vi "NewChoosePass.vi"(1 "IA State Input":T1={"our_robots"=[], "enemy_robots"=[], "balls"=[], "geometry"={"line_width"=0, "field_length"=0, "field_width"=0, "boundary_width"=0, "referee_width"=0, "goal_width"=0, "goal_depth"=0, "goal_wall_width"=0, "center_circle_radius"=0, "defense_radius"=0, "defense_stretch"=0, "free_kick_from_defense_dist"=0, "penalty_spot_from_field_line_dist"=0, "penalty_line_from_spot_dist"=0}, "IA Judge"={"stage"="", "command"="", "our_goalie_id"=0.0, "enemy_goalie_id"=0.0, "command enum"=enum."Halt", "Time"=enum."Azul"}, "Received Timestamp"=timestamp(0 s since 1904-01-01), "Events"={"Touch"=FALSE, "Ball out"=FALSE, "id touch"=0.0, "Ball out of \nVision"=FALSE, "Ball inside \nGoalie area"=FALSE, "Robot not responding"=FALSE, "Robots responding status"=[1.0, 1.0, 1.0, 1.0, 1.0, 1.0], "Enemy Ball \nPossession"=FALSE, "Pass State"=FALSE, "id end of pass"=0.0, "Kick"=FALSE, "Id ini Possession"=0.0, "Ball Possesion"=FALSE, "Id Possesion"=0.0, "Direct Kick"=FALSE, "2nd Strk Ativo"=FALSE}}) -> (0 "Receptor passe":enum16{"Auto", "2nd Striker", "Striker"}(ring))   [LabVIEW 2018]
uses:
  newpass/SSLView/Core/AI Input.ctl
  newpass/SSLView/Core/AI Robot.ctl
  newpass/SSLView/Intel/Functions Enum.ctl
  newpass/SSLView/Intel/AttackerStates.ctl
  newpass/SSLView/Path Planning/RRT/PathDests.ctl
  newpass/SSLView/Path Planning/RRT/PathDest.ctl
  newpass/SSLView/Core/AI Ball.ctl
  newpass/SSLView/Core/Field Size.ctl
  newpass/SSLView/Core/AI Judge.ctl
  newpass/SSLView/Intel/Command Enum.ctl
  newpass/SSLView/Util/Events/Events.ctl
panel:
  in  "x":dbl format="%#_13g"
  in  "y 3":dbl=0.4 format="%#_13g"
  in  "y 2":dbl=0.3 format="%#_13g"
  in  "y":dbl=0.3 format="%#_13g"
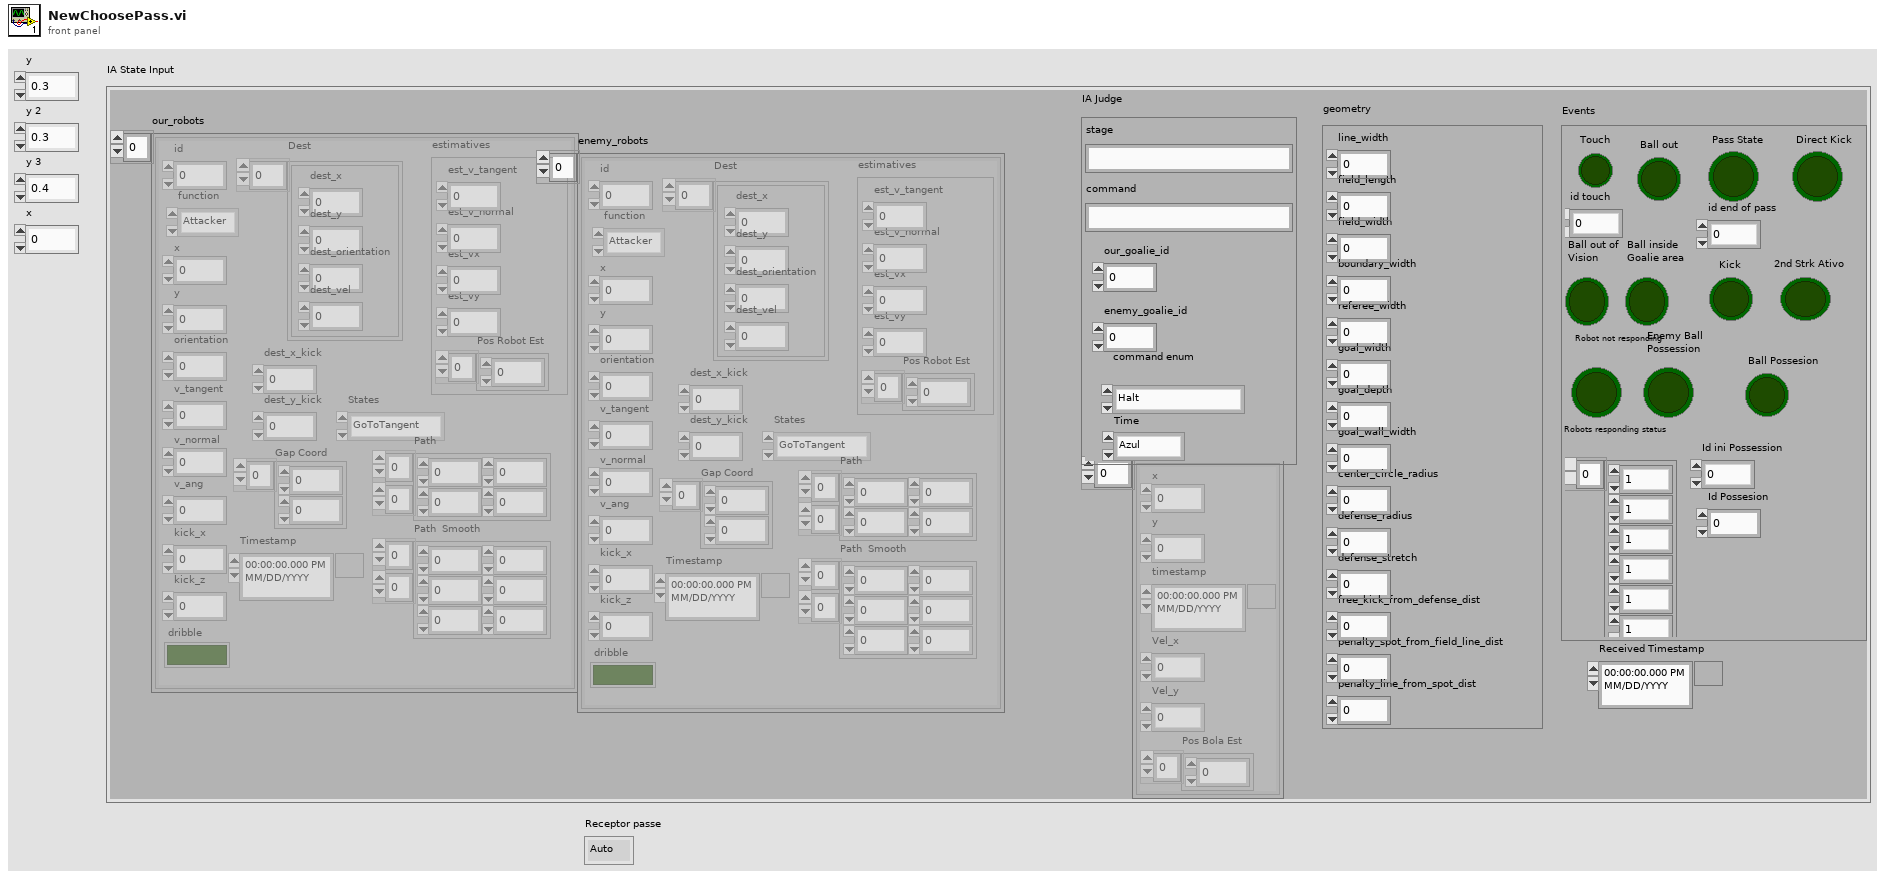
[diagram p1: front panel]
types:
  T1 = typedef "AI Input.ctl" = cluster{"our_robots":T2[], "enemy_robots":T2[], "balls":T7[], "geometry":T8, "IA Judge":T9, "Received Timestamp":timestamp, "Events":T11}
  T2 = typedef "AI Robot.ctl" = cluster{"id":u32, "function":T3, "x":dbl, "y":dbl, "orientation":dbl, "v_tangent":dbl, "v_normal":dbl, "v_ang":dbl, "kick_x":dbl, "kick_z":dbl, "dribble":bool, "Timestamp":timestamp, "estimatives":cluster{"est_v_tangent":dbl, "est_v_normal":dbl, "est_vx":dbl, "est_vy":dbl, "Pos Robot Est":dbl[]}, "dest_x_kick":dbl, "dest_y_kick":dbl, "Gap Coord":dbl[], "States":T4, "Path ":dbl[][], "Path  Smooth":dbl[][], "Dest":T5}
  T3 = typedef "Functions Enum.ctl" = enum16{"2nd Striker", "Attacker", "Goalie", "Defender", "Striker", "Goto 0", "Dummy", "Kicker", "ZigZag 0", "ZigZag 1", "ZigZag 2", "ZigZag 3", "ZigZag 4", "ZigZag 5", "ZigZag 6", "ZigZag 7", "ZigZag 8", ""}
  T4 = typedef "AttackerStates.ctl" = enum16{"Pass", "GoToTangent", "BallGetting", "GoToKick", ""}
  T5 = typedef "PathDests.ctl" = T6[]
  T6 = typedef "PathDest.ctl" = cluster{"dest_x":dbl, "dest_y":dbl, "dest_orientation":dbl, "dest_vel":dbl}
  T7 = typedef "AI Ball.ctl" = cluster{"x":dbl, "y":dbl, "timestamp":timestamp, "Vel_x":dbl, "Vel_y":dbl, "Pos Bola Est":dbl[]}
  T8 = typedef "Field Size.ctl" = cluster{"line_width":u32, "field_length":u32, "field_width":u32, "boundary_width":u32, "referee_width":u32, "goal_width":u32, "goal_depth":u32, "goal_wall_width":u32, "center_circle_radius":u32, "defense_radius":u32, "defense_stretch":u32, "free_kick_from_defense_dist":u32, "penalty_spot_from_field_line_dist":u32, "penalty_line_from_spot_dist":u32}
  T9 = typedef "AI Judge.ctl" = cluster{"stage":string, "command":string, "our_goalie_id":dbl, "enemy_goalie_id":dbl, "command enum":T10, "Time":enum16{"Azul", "Amarelo"}}
  T10 = typedef "Command Enum.ctl" = enum16{"Halt", "Stop", "Force Start", "PKA Normal Start", "Prepare Kickoff Ally", "PKE Normal Start", "Prepare Kickoff Enemy", "Prepare Penalty Ally", "PPA Normal Start", "Prepare Penalty Enemy", "PPE Normal Start", "Direct Free Enemy", "Direct Free Ally", "Indirect Free Enemy", "Indirect Free Ally", "Timeout Enemy", "Timeout Ally", "Goal Enemy", "Goal Ally", "Ball Placement Enemy", "Ball Placement Ally", "Normal Half Time", "Extra Time Break", "Extra Half Time", "None", "Post Game"}
  T11 = typedef "Events.ctl" = cluster{"Touch":bool, "Ball out":bool, "id touch":dbl, "Ball out of \nVision":bool, "Ball inside \nGoalie area":bool, "Robot not responding":bool, "Robots responding status":dbl[], "Enemy Ball \nPossession":bool, "Pass State":bool, "id end of pass":dbl, "Kick":bool, "Id ini Possession":dbl, "Ball Possesion":bool, "Id Possesion":dbl, "Direct Kick":bool, "2nd Strk Ativo":bool}
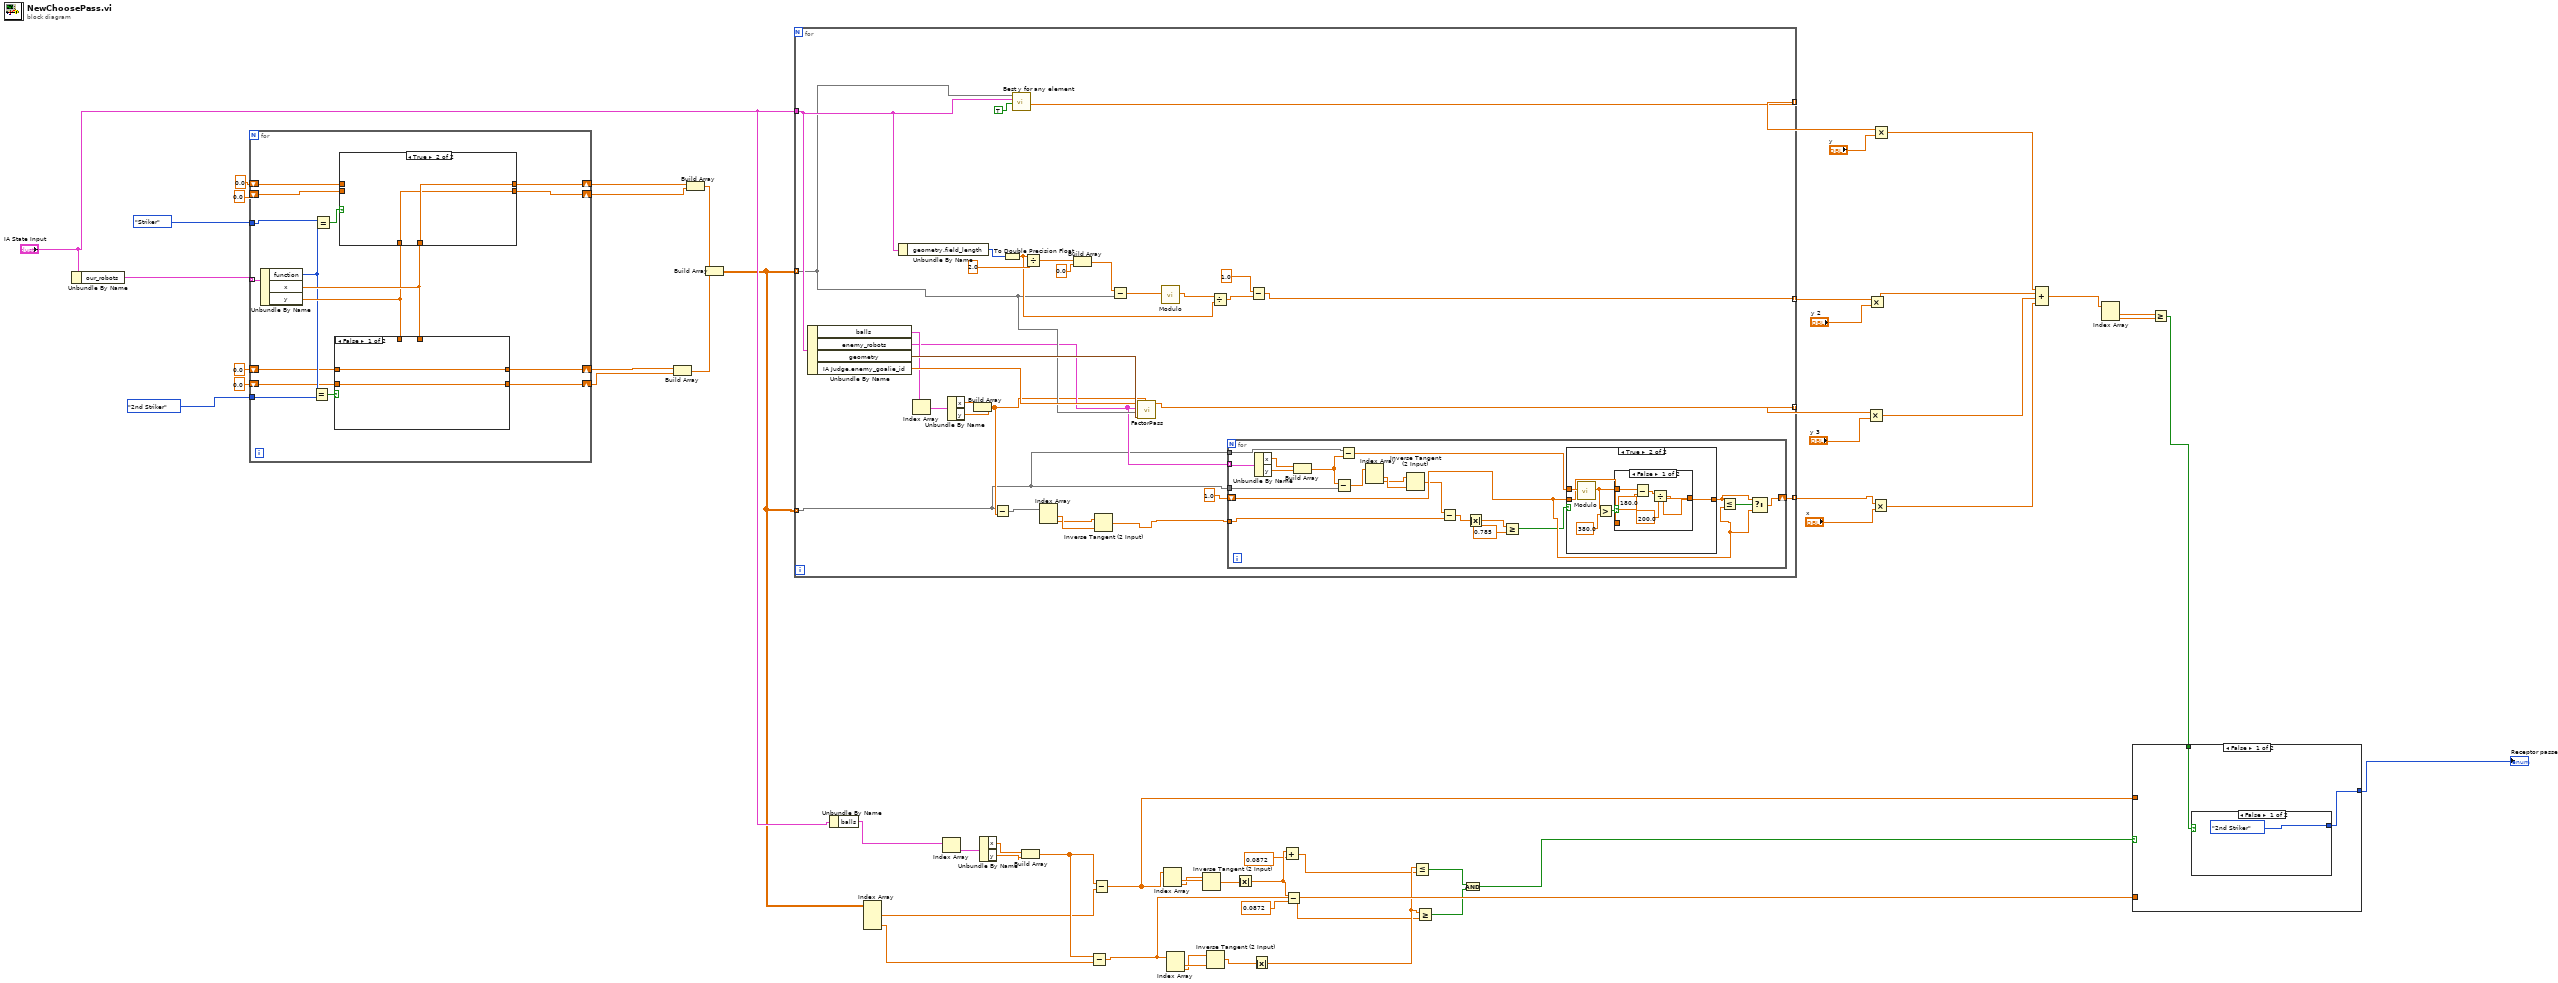
[diagram p0: block diagram]
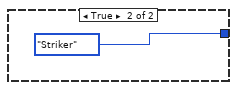
[diagram p2: hidden frame]
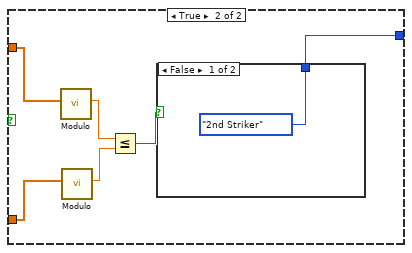
[diagram p3: hidden frame]
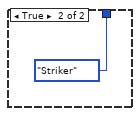
[diagram p4: hidden frame]
diagram:
  n1 = Unbundle By Name("IA State Input") -> ("our_robots"=w56:T2[])
  n2 = for {
    tunnel: w56 -> [w72] mode=indexing
    tunnel: Functions_Enum."Striker" ("y") -> [w65]
    tunnel: Functions_Enum."2nd Striker" ("y") -> [w67]
    shift-right: [w64] -> w51
    shift-left: 0.0 ("x") -> [w63]
    shift-right: [w62] -> w50
    shift-left: 0.0 ("y") -> [w61]
    shift-right: [w59] -> w46
    shift-left: 0.0 ("y") -> [w57]
    shift-right: [w60] -> w47
    shift-left: 0.0 ("x") -> [w58]
    n3 = Unbundle By Name(w72) -> ("function"=w66:T3, "x"=w71:dbl, "y"=w70:dbl)
    n4 = Equal?(x=w66, y=w67) -> (x = y?=w68:bool)
    n5 = Equal?(x=w65, y=w66) -> (x = y?=w69:bool)
    n6 = case shown="False" w68 {
      tunnel: w71 -> [_ w76]
      tunnel: w70 -> [_ w75]
      tunnel: [w74 w76] -> w64
      tunnel: w63 -> [w74 _]
      tunnel: [w73 w75] -> w62
      tunnel: w61 -> [w73 _]
      frame False {
      }
      frame True {
      }
    }
    n7 = case shown="True" w69 {
      tunnel: w71 -> [_ w80]
      tunnel: w70 -> [_ w79]
      tunnel: [w78 w80] -> w60
      tunnel: [w77 w79] -> w59
      tunnel: w58 -> [w78 _]
      tunnel: w57 -> [w77 _]
      frame False {
      }
      frame True {
      }
    }
  }
  n8 = Build Array(w51, w50) -> (w54:dbl[])
  n9 = Build Array(w47, w46) -> (w55:dbl[])
  n10 = Build Array(w55, w54) -> (w4:dbl[][])
  n11 = for {
    tunnel: w4 -> [w90] mode=indexing
    tunnel: "IA State Input" -> [w99]
    tunnel: [w100] -> w43 mode=indexing
    tunnel: [w93] -> w42 mode=indexing
    tunnel: [w92] -> w41 mode=indexing
    tunnel: w4 -> [w83] mode=indexing
    tunnel: [w86] -> w3 mode=indexing
    n12 = Unbundle By Name(w99) -> ("balls"=w91:T7[], "enemy_robots"=w88:T2[], "geometry"=w95:T8, "IA Judge.enemy_goalie_id"=w94:dbl)
    n13 = Unbundle By Name(w99) -> ("geometry.field_length"=w110:u32)
    n14 = Index Array(array=w91) -> (element=w98:T7)  [unwired: 1 in]
    n15 = Unbundle By Name(w98) -> ("x"=w97:dbl, "y"=w96:dbl)
    n16 = Build Array(w97, w96) -> (w85:dbl[])
    n17 = Subtract(x=w83, y=w85) -> (x-y=w89:dbl[])
    n18 = To Double Precision Float(number=w110) -> (double precision float=w103:dbl)
    n19 = call "Best y for any element.vi"("Maior intervalo(T)\nMaior angulo(F)"=TRUE ("Maior intervalo(T)\nMaior angulo(F)"), "IA State"=w99, "Element Position"=w90) -> ("Goal Gap Normalizado(%do gol aberta)"=w100:dbl)  [unwired: 4 in, 4 out]
    n20 = Divide(x=w103, y=2.0) -> (x/y=w108:dbl)
    n21 = Index Array(array=w89) -> (element #1=w82:dbl, element #2=w81:dbl)  [unwired: 2 in]
    n22 = Build Array(w108, 0.0 ("element")) -> (w107:dbl[])
    n23 = Inverse Tangent (2 Input)(1:w82, 2:w81) -> (0:w84:dbl)
    n24 = Subtract(x=w107, y=w90) -> (x-y=w105:dbl[])
    n25 = call "FactorPass.vi"("Coordenada bola"=w85, "geometry"=w95, "Coordenada robo"=w90, "enemy_robots"=w88, "enemy_goalie_id"=w94) -> ("Critério de marcação Normalizado"=w92:dbl)  [unwired: 6 out]
    n26 = call "Modulo.vi"("2D vector"=w105) -> ("Modulo"=w104:dbl)  [unwired: 10 in]
    n27 = Divide(x=w104, y=w103) -> (x/y=w101:dbl)
    n28 = for {
      tunnel: w88 -> [w131] mode=indexing
      tunnel: w84 -> [w119]
      tunnel: w83 -> [w129]
      shift-right: [w123] -> w86
      shift-left: 1.0 ("x") -> [w124]
      tunnel: w83 -> [w127]
      n29 = Unbundle By Name(w131) -> ("x"=w120:dbl, "y"=w121:dbl)
      n30 = Build Array(w120, w121) -> (w128:dbl[])
      n31 = Subtract(x=w128, y=w129) -> (x-y=w130:dbl[])
      n32 = Subtract(x=w127, y=w128) -> (x-y=w126:dbl[])
      n33 = Index Array(array=w130) -> (element #1=w113:dbl, element #2=w112:dbl)  [unwired: 2 in]
      n34 = Inverse Tangent (2 Input)(1:w113, 2:w112) -> (0:w118:dbl)
      n35 = Subtract(x=w118, y=w119) -> (x-y=w117:dbl)
      n36 = Absolute Value(x=w117) -> (abs(x)=w116:dbl)
      n37 = Greater Or Equal?(x=w116, y=0.785) -> (x >= y?=w115:bool)
      n38 = case shown="True" w115 {
        tunnel: w126 -> [_ w138]
        tunnel: w124 -> [w132 w135]
        tunnel: [w132 w134] -> w125
        frame False {
        }
        frame True {
          n39 = call "Modulo.vi"("2D vector"=w138) -> ("Modulo"=w133:dbl)  [unwired: 10 in]
          n40 = Greater?(x=w133, y=380.0) -> (0:w136:bool)
          n41 = case shown="False" w136 {
            tunnel: w135 -> [_ w144]
            tunnel: [w143 w144] -> w134
            tunnel: w133 -> [w142 _]
            frame False {
              n42 = Subtract(x=w142, y=180.0) -> (x-y=w140:dbl)
              n43 = Divide(x=w140, y=200.0) -> (x/y=w143:dbl)
            }
            frame True {
            }
          }
        }
      }
      n44 = Less Or Equal?(x=w125, y=w124) -> (x <= y?=w122:bool)
      n45 = Select(t=w125, s=w122, f=w124) -> (s? t:f=w123:dbl)
    }
    n46 = Subtract(x=1.0, y=w101) -> (x-y=w93:dbl)
  }
  n47 = Unbundle By Name("IA State Input") -> ("balls"=w10:T7[])
  n48 = Index Array(array=w4) -> (element #1=w6:dbl[], element #2=w5:dbl[])  [unwired: 4 in]
  n49 = Index Array(array=w10) -> (element=w11:T7)  [unwired: 1 in]
  n50 = Unbundle By Name(w11) -> ("x"=w12:dbl, "y"=w13:dbl)
  n51 = Build Array(w12, w13) -> (w29:dbl[])
  n52 = Subtract(x=w29, y=w5) -> (x-y=w30:dbl[])
  n53 = Subtract(x=w29, y=w6) -> (x-y=w31:dbl[])
  n54 = Index Array(array=w31) -> (element #1=w15:dbl, element #2=w14:dbl)  [unwired: 2 in]
  n55 = Index Array(array=w30) -> (element #1=w19:dbl, element #2=w18:dbl)  [unwired: 2 in]
  n56 = Inverse Tangent (2 Input)(1:w15, 2:w14) -> (0:w20:dbl)
  n57 = Inverse Tangent (2 Input)(1:w19, 2:w18) -> (0:w22:dbl)
  n58 = Absolute Value(x=w20) -> (abs(x)=w21:dbl)
  n59 = Absolute Value(x=w22) -> (abs(x)=w25:dbl)
  n60 = Add(x=w21, y=0.0872) -> (x+y=w23:dbl)
  n61 = Subtract(x=w21, y=0.0872) -> (x-y=w24:dbl)
  n62 = Less Or Equal?(x=w25, y=w23) -> (x <= y?=w26:bool)
  n63 = Greater Or Equal?(x=w25, y=w24) -> (x >= y?=w27:bool)
  n64 = And(x=w26, y=w27) -> (x .and. y?=w28:bool)
  n65 = Multiply(x=w41, y="y 3") -> (x*y=w35:dbl[])
  n66 = Multiply(x=w42, y="y 2") -> (x*y=w36:dbl[])
  n67 = Multiply(x=w3, y="x") -> (x*y=w1:dbl[])
  n68 = Multiply(x=w43, y="y") -> (x*y=w37:dbl[])
  n69 = Compound Arithmetic op=ADD(w37, w36, w35, w1) -> (w34:dbl[])
  n70 = Index Array(array=w34) -> (element #1=w33:dbl, element #2=w32:dbl)  [unwired: 2 in]
  n71 = Greater Or Equal?(x=w33, y=w32) -> (x >= y?=w8:bool)
  n72 = case shown="False" w28 {
    tunnel: w30 -> [_ w153]
    tunnel: w31 -> [_ w154]
    tunnel: [w146 w149] -> w7
    tunnel: w8 -> [w145 _]
    frame False {
      n73 = case shown="False" w145 {
        tunnel: [enum16{"Auto", "2nd Striker", "Striker"}."2nd Striker" ("Receptor passe") enum16{"Auto", "2nd Striker", "Striker"}."Striker" ("Receptor passe")] -> w146
        frame False {
        }
        frame True {
        }
      }
    }
    frame True {
      n74 = call "Modulo.vi"("2D vector"=w154) -> ("Modulo"=w152:dbl)  [unwired: 10 in]
      n75 = call "Modulo.vi"("2D vector"=w153) -> ("Modulo"=w151:dbl)  [unwired: 10 in]
      n76 = Less Or Equal?(x=w152, y=w151) -> (x <= y?=w150:bool)
      n77 = case shown="False" w150 {
        tunnel: [enum16{"Auto", "2nd Striker", "Striker"}."2nd Striker" ("Receptor passe") enum16{"Auto", "2nd Striker", "Striker"}."Striker" ("Receptor passe")] -> w149
        frame False {
        }
        frame True {
        }
      }
    }
  }
  "Receptor passe" <- w7
